vi "2DSmooth(SubVI).vi"(10 "Input array":dbl[][](array[numeric]), 11 "Interpolation factor":i32=10) -> (3 "Array":dbl[][](array[numeric]))   [LabVIEW 2014]
uses:
  <vilib>/Analysis/NI_AALPro.lvlib
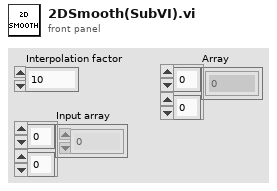
[diagram p1: front panel]
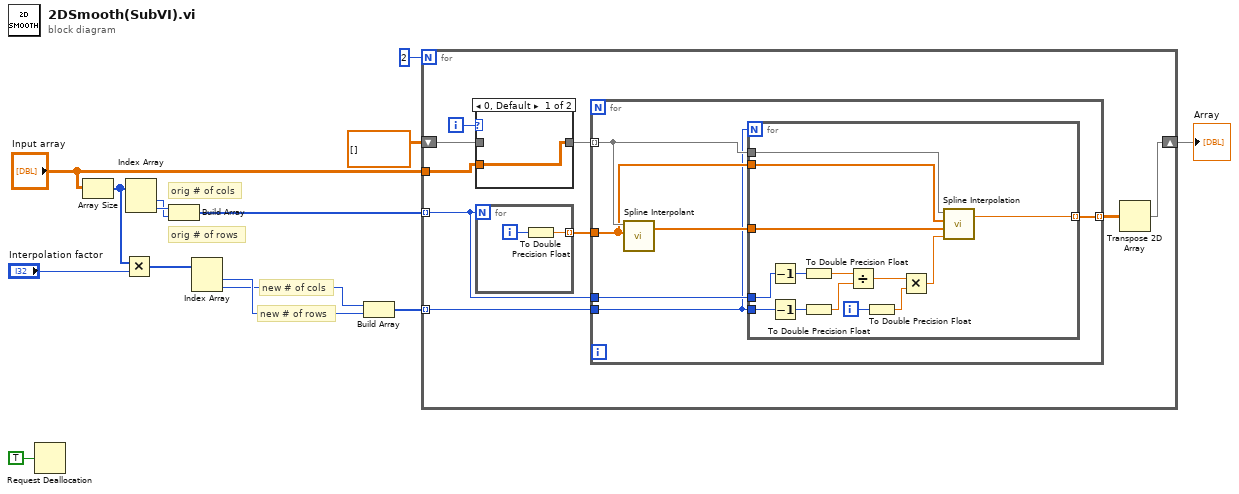
[diagram p0: block diagram]
diagram:
  # "new # of rows"
  # "new # of cols"
  # "orig # of rows"
  # "orig # of cols"
  n1 = Request Deallocation(TRUE ("flag")) -> ()
  n2 = Array Size(array="Input array") -> (size(s)=w10:i32[])
  n3 = Multiply(x=w10, y="Interpolation factor") -> (x*y=w8:i32[])
  n4 = Index Array(array=w10) -> (element #1=w13:i32, element #2=w14:i32)  [unwired: 2 in]
  n5 = Build Array(w14, w13) -> (w4:i32[])
  n6 = Index Array(array=w8) -> (element #1=w12:i32, element #2=w11:i32)  [unwired: 2 in]
  n7 = Build Array(w11, w12) -> (w3:i32[])
  n8 = for {
    N: 2 -> [_]
    tunnel: "Input array" -> [w19]
    tunnel: w4 -> [w21] mode=indexing
    shift-right: [w15] -> w7
    shift-left: dbl[][] [] -> [w17]
    tunnel: w3 -> [w16] mode=indexing
    i -> [w20]
    n9 = case shown="0, Default" w20 {
      tunnel: w19 -> [w24 _]
      tunnel: [w24 w25] -> w18
      tunnel: w17 -> [_ w25]
      frame 0, Default {
      }
      frame 1 {
      }
    }
    n10 = for {
      N: w21 -> [_]
      tunnel: [w26] -> w23 mode=indexing
      i -> [w27]
      n11 = To Double Precision Float(number=w27) -> (double precision float=w26:dbl)
    }
    n12 = for {
      tunnel: w21 -> [w33]
      tunnel: w18 -> [w31] mode=indexing
      tunnel: w23 -> [w30]
      tunnel: [w29] -> w22 mode=indexing
      tunnel: w16 -> [w28]
      n13 = call <vilib>:"Spline Interpolant.vi"("X"=w30, "Y"=w31) -> ("Interpolant"=w32:dbl[])  [unwired: 2 in, 1 out]
      n14 = for {
        N: w28 -> [_]
        tunnel: w33 -> [w44]
        tunnel: w32 -> [w42]
        tunnel: w31 -> [w41]
        tunnel: w30 -> [w40]
        tunnel: [w39] -> w29 mode=indexing
        tunnel: w28 -> [w37]
        i -> [w43]
        n15 = Decrement(x=w44) -> (x-1=w47:i32)
        n16 = Decrement(x=w37) -> (x-1=w46:i32)
        n17 = To Double Precision Float(number=w47) -> (double precision float=w35:dbl)
        n18 = To Double Precision Float(number=w46) -> (double precision float=w34:dbl)
        n19 = Divide(x=w35, y=w34) -> (x/y=w45:dbl)
        n20 = To Double Precision Float(number=w43) -> (double precision float=w36:dbl)
        n21 = Multiply(x=w45, y=w36) -> (x*y=w38:dbl)
        n22 = call <vilib>:"Spline Interpolation.vi"("x value"=w38, "Interpolant"=w42, "X"=w40, "Y"=w41) -> ("interpolation value"=w39:dbl)  [unwired: 1 out]
      }
    }
    n23 = Transpose 2D Array(2D array=w22) -> (transposed array=w15:dbl[][])
  }
  "Array" <- w7
